vi "Initialize Subpanel Objects.vi"(8 "error in (no error)":errorcluster, 10 "SubPanelRefs":refnum<vi>[](array[refnum]), 11 "HSplitted in":refnum<class "HSplitted.lvclass">) -> (0 "error out":errorcluster, 3 "HSplitted out":refnum<class "HSplitted.lvclass">)   [LabVIEW 2020, in "HSplitted.lvlib" / "HSplitted.lvclass"]
uses:
  HSplitted.lvclass
  HSplitted.lvclass/HSplitted.ctl
  <vilib>/MGI/Panel Manager/Panel/Panel.lvlib
  <vilib>/MGI/Panel Manager/Panel/Panel/Subpanel/Subpanel.vi
  <vilib>/MGI/Panel Manager/Panel/Panel/Subpanel/Subpanel.lvclass
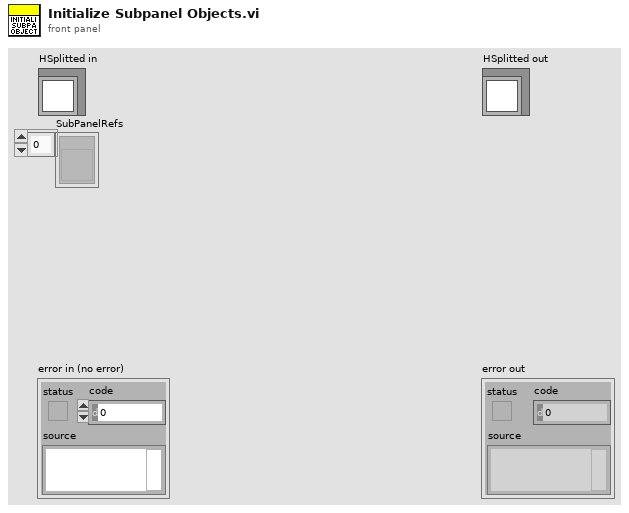
[diagram p1: front panel]
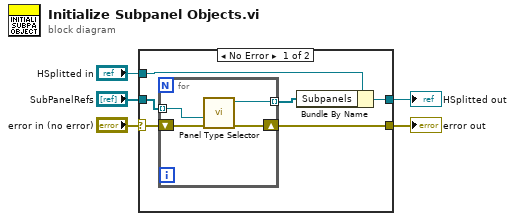
[diagram p0: block diagram]
diagram:
  n1 = case shown="No Error" "error in (no error)" {
    selector: "error in (no error)" -> [w10 w17]
    tunnel: [w6 w17] -> w4
    tunnel: [w8 w16] -> w2
    tunnel: "HSplitted in" -> [w9 w16]
    tunnel: "SubPanelRefs" -> [w7 _]
    frame No Error {
      n2 = for {
        tunnel: [w15] -> w11 mode=indexing
        shift-right: [w13] -> w6
        shift-left: w10 -> [w14]
        tunnel: w7 -> [w12] mode=indexing
        n3 = call-poly <vilib>:"Panel Type Selector.vi"("Error In"=w14, "Sub Panel"=w12) -> ("Error Out"=w13:errorcluster, "Subpanel Out"=w15:refnum<class "Subpanel.lvclass">)  [unwired: 8 in]
      }
      n4 = Bundle By Name(cluster=w9, "Subpanels"=w11) -> (w8:refnum<class "HSplitted.lvclass">)
    }
    frame Error {
    }
  }
  "error out" <- w4
  "HSplitted out" <- w2
